vi "KE622x -- 2182 -A A Read-Out.vi"(0 "622x Resource In":refnum<visa-resource-name>, 1 "Check For SCPI Errors? (T)":bool=TRUE, 7 "Time of one measurement":dbl=1000.0 min=0.0, 11 "error in (no error)":errorcluster) -> (4 "622x Resource Out (dupl)":refnum<visa-resource-name>, 8 "2182-A Reponse String":string, 15 "error out":errorcluster)   [LabVIEW 2013, in "Keithly user program.lvlib"]
doc: "Return measured value from instrument KE2182-A."
uses:
  Keithly user program.lvlib
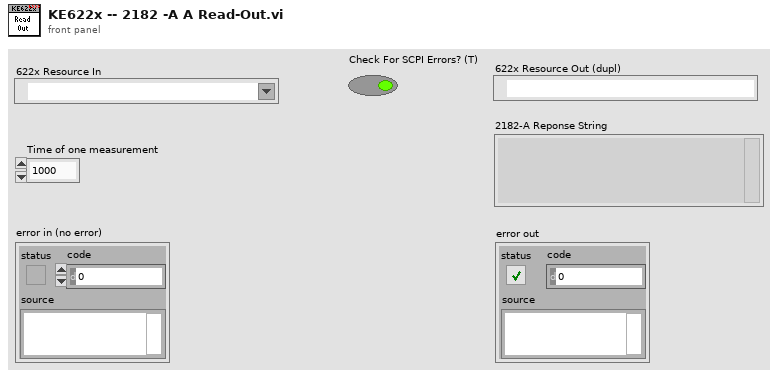
[diagram p1: front panel]
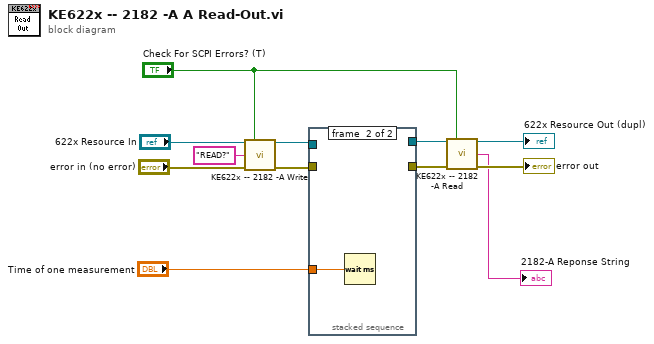
[diagram p0: block diagram]
diagram:
  n1 = call "KE622x -- 2182 -A Write.vi"("Resource In"="622x Resource In", "Check For SCPI Errors? (T)"="Check For SCPI Errors? (T)", "2182-A Write String"="READ?", "error in (no error)"="error in (no error)") -> ("Resource Out (dupl)"=w10:refnum<visa-resource-name>, "error out"=w9:errorcluster)  [unwired: 10 in]
  n2 = stacked-sequence {
    tunnel: w9 -> [w14 _]
    tunnel: [w14 _] -> w7
    tunnel: [w13 _] -> w8
    tunnel: w10 -> [w13 _]
    tunnel: "Time of one measurement" -> [_ w15]
    frame #0 {
    }
    frame #1 {
      n3 = Wait (ms)(milliseconds to wait=w15) -> ()  [unwired: 1 out]
    }
  }
  n4 = call "KE622x -- 2182 -A Read.vi"("622x Resource In"=w8, "Check For SCPI Errors? (T)"="Check For SCPI Errors? (T)", "error in (no error)"=w7) -> ("622x Resource Out (dupl)"=→"622x Resource Out (dupl)":refnum<visa-resource-name>, "2182-A Reponse String"=→"2182-A Reponse String":string, "error out"=→"error out":errorcluster)  [unwired: 10 in]
